vi "QR_Printer.vi"(3 "GetBIM 4":T1={"xPosition"="9", "yPosition"="2", "familyName"="Arial", "emSize"=6.0, "printText"="CS-RX110JHA2"}, 4 "QRC":T3={"startX"="2", "startY"="3", "cellSize"=3, "inoutMode"=1, "maskNumber"=9, "errorLevel"=1, "terminator"=2, "modelNumber"=2, "strData"="設定機種品番"} {"terminator" items=["NUL"=1, "ETX"=2, "EOT"=3]}, 5 "GetBIM 2":T1={"xPosition"="9", "yPosition"="2", "familyName"="Arial", "emSize"=6.0, "printText"="CS-RX110JHA2"}, 6 "GetBIM 3":T1={"xPosition"="9", "yPosition"="2", "familyName"="Arial", "emSize"=6.0, "printText"="CS-RX110JHA2"}, 7 "GetBIM 1":T1={"xPosition"="9", "yPosition"="2", "familyName"="Arial", "emSize"=6.0, "printText"="CS-RX110JHA2"}, 8 "error in (no error)":errorcluster, 9 "PRT":T2={"quantity"=1, "cutUnit"=0, "fixedNO"=1}, 10 "FMT":T4={"formatNo"=1, "x"="25", "y"="10", "Is180Rotation"=FALSE, "IsReflected"=0, "copies"=1}, 11 "printName":string="Ring 412PEI+") -> (0 "error out":errorcluster)   [LabVIEW 2014]
uses:
  controls/FMT.ctl
  controls/GetBIM.ctl
  controls/QRC.ctl
  controls/PRT.ctl
  System.Drawing
  C:/AC-BarCode/SDK_v1.3.2.0/RingPrinter.dll
  SDK_v1.3.2.0/RingPrinter.dll
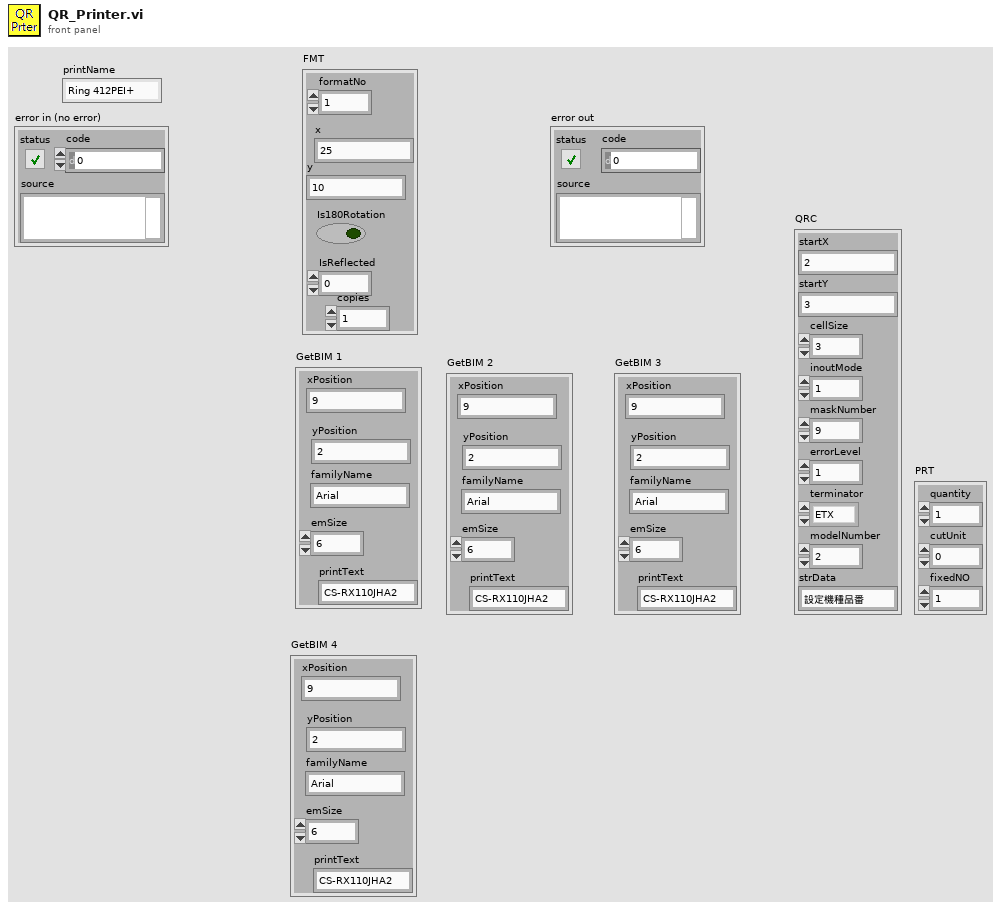
[diagram p1: front panel]
types:
  T1 = typedef "GetBIM.ctl" = cluster{"xPosition":string, "yPosition":string, "familyName":string, "emSize":sgl, "printText":string}
  T2 = typedef "PRT.ctl" = cluster{"quantity":i32, "cutUnit":i32, "fixedNO":i32}
  T3 = typedef "QRC.ctl" = cluster{"startX":string, "startY":string, "cellSize":i32, "inoutMode":i32, "maskNumber":i32, "errorLevel":i32, "terminator":i32, "modelNumber":i32, "strData":string}
  T4 = typedef "FMT.ctl" = cluster{"formatNo":i32, "x":string, "y":string, "Is180Rotation":bool, "IsReflected":u8, "copies":u8}
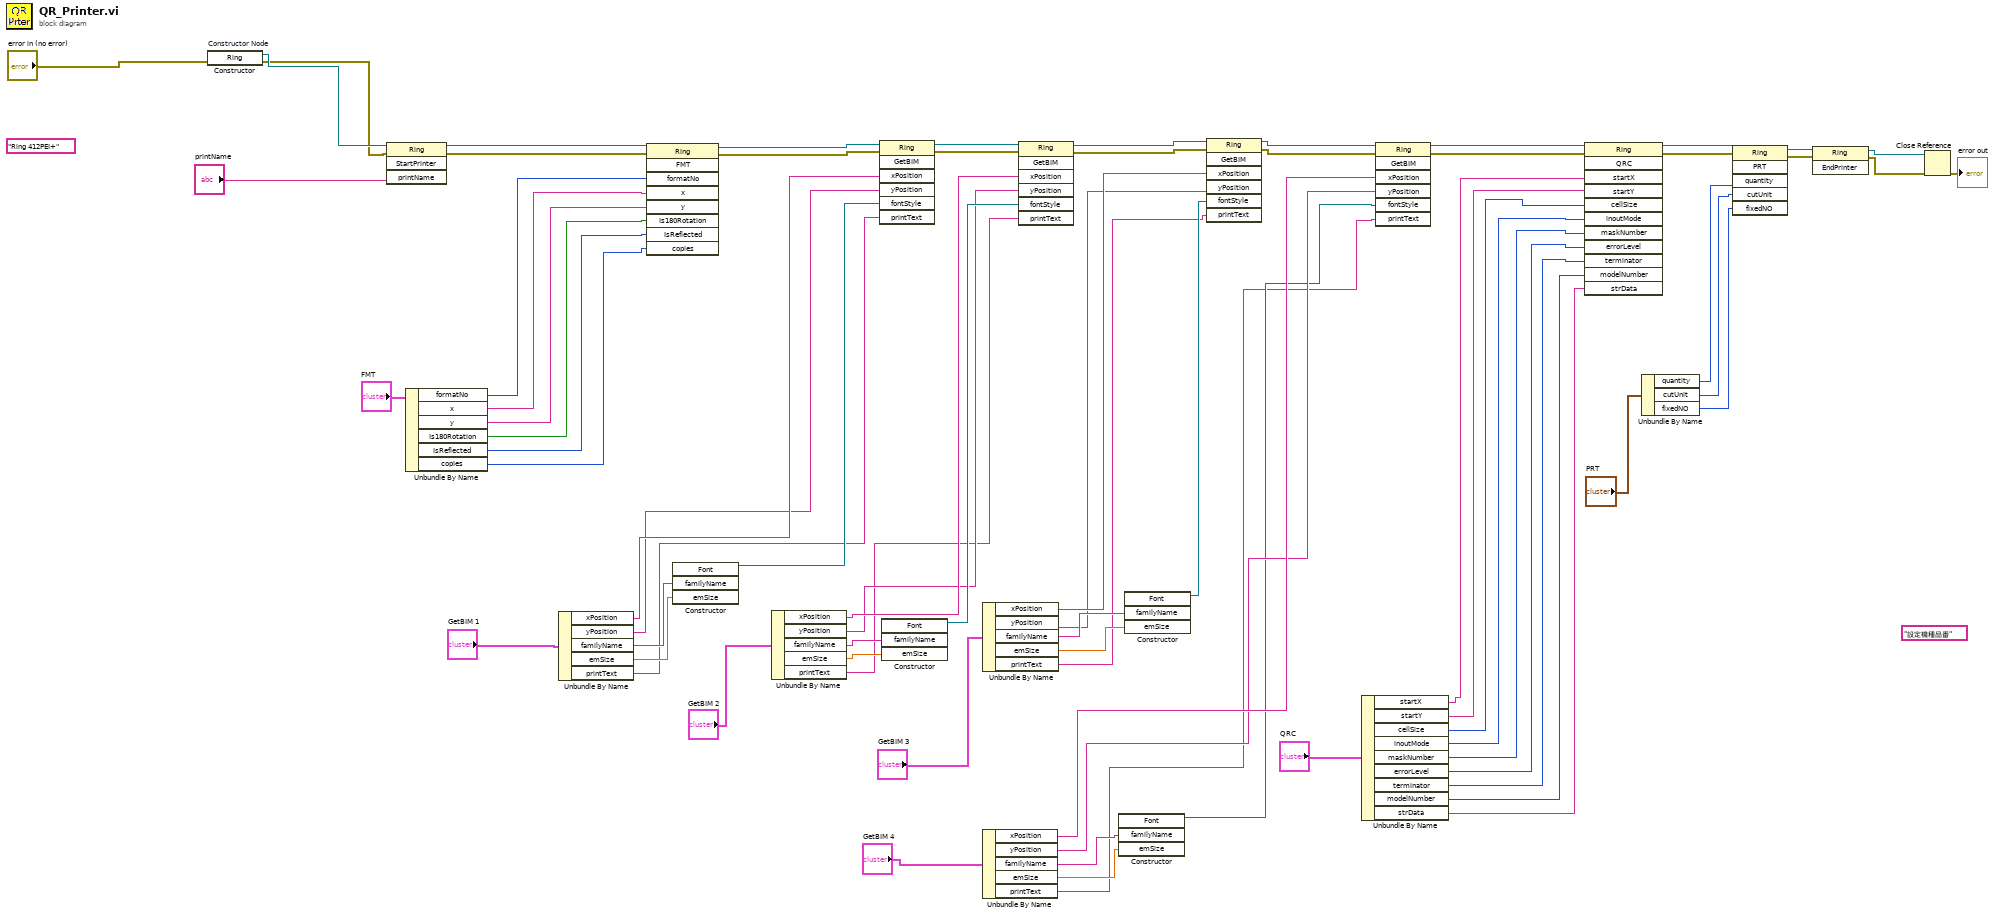
[diagram p0: block diagram]
diagram:
  (unwired) "Ring 412PEI+" ("printName")
  (unwired) "設定機種品番" ("strData")
  n1 = constructor on="Constructor Node" class="Ring"(error in="error in (no error)") -> (reference out=w72:refnum<k24>, error out=w56:errorcluster)  [unwired: 2 in, 1 out]
  n2 = invoke class="Ring" method="StartPrinter"(reference=w72, error in=w56, "printName"="printName") -> (reference out=w71:refnum<k24>, error out=w70:errorcluster)  [unwired: 1 in, 2 out]
  n3 = Unbundle By Name("FMT") -> ("formatNo"=w17:i32, "x"=w16:string, "y"=w15:string, "Is180Rotation"=w14:bool, "IsReflected"=w13:u8, "copies"=w12:u8)
  n4 = Unbundle By Name("GetBIM 1") -> ("xPosition"=w21:string, "yPosition"=w20:string, "familyName"=w24:string, "emSize"=w23:sgl, "printText"=w19:string)
  n5 = invoke class="Ring" method="FMT"(reference=w71, error in=w70, "formatNo"=w17, "x"=w16, "y"=w15, "Is180Rotation"=w14, "IsReflected"=w13, "copies"=w12) -> (reference out=w61:refnum<k24>, error out=w60:errorcluster)  [unwired: 1 in, 7 out]
  n6 = constructor class="Font"("familyName"=w24, "emSize"=w23) -> (reference out=w22:refnum<k24>)  [unwired: 3 in, 4 out]
  n7 = Unbundle By Name("GetBIM 2") -> ("xPosition"=w28:string, "yPosition"=w27:string, "familyName"=w31:string, "emSize"=w30:sgl, "printText"=w26:string)
  n8 = invoke class="Ring" method="GetBIM"(reference=w61, error in=w60, "xPosition"=w21, "yPosition"=w20, "fontStyle"=w22, "printText"=w19) -> (reference out=w63:refnum<k24>, error out=w62:errorcluster)  [unwired: 1 in, 5 out]
  n9 = constructor class="Font"("familyName"=w31, "emSize"=w30) -> (reference out=w29:refnum<k24>)  [unwired: 3 in, 4 out]
  n10 = Unbundle By Name("GetBIM 4") -> ("xPosition"=w4:string, "yPosition"=w3:string, "familyName"=w6:string, "emSize"=w5:sgl, "printText"=w1:string)
  n11 = Unbundle By Name("GetBIM 3") -> ("xPosition"=w35:string, "yPosition"=w34:string, "familyName"=w37:string, "emSize"=w36:sgl, "printText"=w33:string)
  n12 = invoke class="Ring" method="GetBIM"(reference=w63, error in=w62, "xPosition"=w28, "yPosition"=w27, "fontStyle"=w29, "printText"=w26) -> (reference out=w59:refnum<k24>, error out=w58:errorcluster)  [unwired: 1 in, 5 out]
  n13 = constructor class="Font"("familyName"=w6, "emSize"=w5) -> (reference out=w2:refnum<k24>)  [unwired: 3 in, 4 out]
  n14 = constructor class="Font"("familyName"=w37, "emSize"=w36) -> (reference out=w38:refnum<k24>)  [unwired: 3 in, 4 out]
  n15 = invoke class="Ring" method="GetBIM"(reference=w59, error in=w58, "xPosition"=w35, "yPosition"=w34, "fontStyle"=w38, "printText"=w33) -> (reference out=w11:refnum<k24>, error out=w10:errorcluster)  [unwired: 1 in, 5 out]
  n16 = Unbundle By Name("QRC") -> ("startX"=w48:string, "startY"=w47:string, "cellSize"=w46:i32, "inoutMode"=w45:i32, "maskNumber"=w44:i32, "errorLevel"=w43:i32, "terminator"=w42:i32, "modelNumber"=w41:i32, "strData"=w40:string)
  n17 = invoke class="Ring" method="GetBIM"(reference=w11, error in=w10, "xPosition"=w4, "yPosition"=w3, "fontStyle"=w2, "printText"=w1) -> (reference out=w9:refnum<k24>, error out=w8:errorcluster)  [unwired: 1 in, 5 out]
  n18 = invoke class="Ring" method="QRC"(reference=w9, error in=w8, "startX"=w48, "startY"=w47, "cellSize"=w46, "inoutMode"=w45, "maskNumber"=w44, "errorLevel"=w43, "terminator"=w42, "modelNumber"=w41, "strData"=w40) -> (reference out=w69:refnum<k24>, error out=w68:errorcluster)  [unwired: 1 in, 10 out]
  n19 = Unbundle By Name("PRT") -> ("quantity"=w52:i32, "cutUnit"=w51:i32, "fixedNO"=w50:i32)
  n20 = invoke class="Ring" method="PRT"(reference=w69, error in=w68, "quantity"=w52, "cutUnit"=w51, "fixedNO"=w50) -> (reference out=w67:refnum<k24>, error out=w66:errorcluster)  [unwired: 1 in, 4 out]
  n21 = invoke class="Ring" method="EndPrinter"(reference=w67, error in=w66) -> (reference out=w65:refnum<k24>, error out=w64:errorcluster)  [unwired: 1 in, 1 out]
  n22 = Close Reference(reference=w65, error in (no error)=w64) -> (error out=→"error out":errorcluster)
